vi "Simple_UP_DWN_Timer.vi"() -> ()   [LabVIEW 2010]
doc: "Simple timer that increments or decrements in seconds.\nDecremented value will not go below zero."
panel:
  out "Running?":bool
  in  "Timer (HH:MM:SS)":string="00:00:00"
  in  "Exit":bool
  in  "Stop":bool
  in  "Start":bool
  in  "Counter Mode":enum32{"Count Up", "Count Down"}(radio)
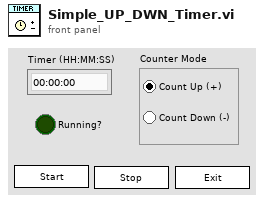
[diagram p1: front panel]
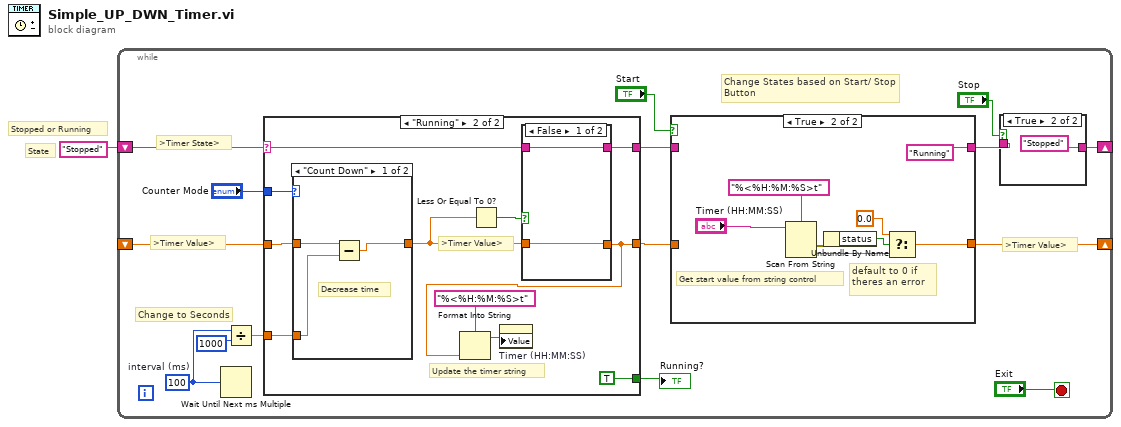
[diagram p0: block diagram]
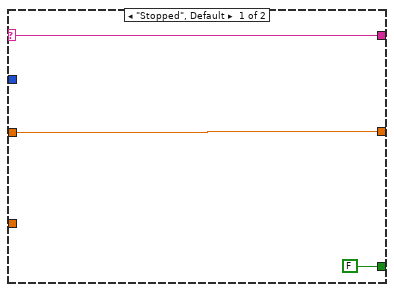
[diagram p4: hidden frame]
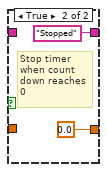
[diagram p5: hidden frame]
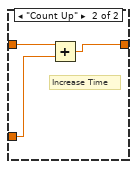
[diagram p6: hidden frame]
diagram:
  # "Stopped or Running"
  # "State"
  n1 = while {
    shift-right: [w10] -> _
    shift-left: "Stopped" -> [w15]
    shift-right: [w9] -> _
    shift-left: _ -> [w8]
    stop <- "Exit" stop-if-true
    w6 = u32 100  # interval (ms)
    # ">Timer Value>"
    # ">Timer Value>"
    # ">Timer State>"
    # "Change to Seconds"
    # "Change States based on Start/ Stop\nButton"
    n2 = Wait Until Next ms Multiple(millisecond multiple=w6) -> ()  [unwired: 1 out]
    n3 = Divide(x=w6, y=u32 1000) -> (x/y=w4:dbl)
    n4 = case shown="\"Running\"" w15 {
      selector: w15 -> [w29 w36]
      tunnel: w8 -> [w31 w41]
      tunnel: "Counter Mode" -> [_ w42]
      tunnel: [w31 w32] -> w7
      tunnel: w4 -> [_ w40]
      tunnel: [FALSE ("Running?") TRUE ("Running?")] -> w3
      tunnel: [w29 w33] -> w2
      frame "Stopped", Default {
      }
      frame "Running" {
        # ">Timer Value>"
        # "Update the timer string"
        n5 = case shown="\"Count Down\"" w42 {
          tunnel: w41 -> [w49 w52]
          tunnel: [w47 w51] -> w35
          tunnel: w40 -> [w48 w50]
          frame "Count Down" {
            # "Decrease time"
            n6 = Subtract(x=w49, y=w48) -> (x-y=w47:dbl)
          }
          frame "Count Up" {
            # "Increase Time"
            n7 = Add(x=w52, y=w50) -> (x+y=w51:dbl)
          }
        }
        n8 = Less Or Equal To 0?(x=w35) -> (x <= 0?=w34:bool)
        n9 = case shown="False" w34 {
          tunnel: w35 -> [w43 _]
          tunnel: [w43 0.0 ("t")] -> w32
          tunnel: w36 -> [w44 _]
          tunnel: [w44 "Stopped"] -> w33
          frame False {
          }
          frame True {
            # "Stop timer when count down reaches 0"
          }
        }
        n10 = Format Into String(format string="%<%H:%M:%S>t", w32) -> (resulting string=w39:string)  [unwired: 2 in, 1 out]
        n11 = property on="Timer (HH:MM:SS)" class="Str"("Value"=w39) -> ()  [unwired: 2 in, 2 out]
      }
    }
    "Running?" <- w3
    n12 = case shown="True" "Start" {
      tunnel: [w20 "Running"] -> w11
      tunnel: w2 -> [w20 _]
      tunnel: [w19 w22] -> w9
      tunnel: w7 -> [w19 _]
      frame False {
      }
      frame True {
        # "default to 0 if theres an error"
        # "Get start value from string control"
        n13 = Scan From String(format string="%<%H:%M:%S>t", input string="Timer (HH:MM:SS)") -> (error out=w25:errorcluster, output 1=w23:dbl)  [unwired: 3 in, 2 out]
        n14 = Unbundle By Name(w25) -> ("status"=w21:bool)
        n15 = Select(t=0.0, s=w21, f=w23) -> (s? t:f=w22:dbl)
      }
    }
    n16 = case shown="True" "Stop" {
      tunnel: [w17 "Stopped"] -> w10
      tunnel: w11 -> [w17 _]
      frame False {
      }
      frame True {
      }
    }
  }
